vi "String Trim Whitespace.vi"(11 "String":string) -> (3 "*(type *) &x":string)   [LabVIEW 2019]
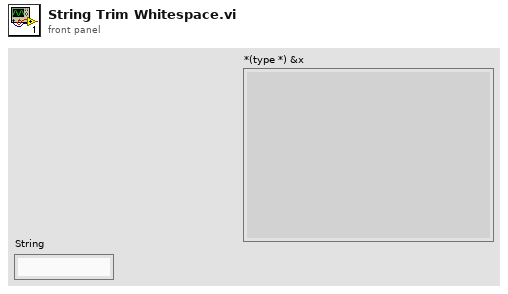
[diagram p1: front panel]
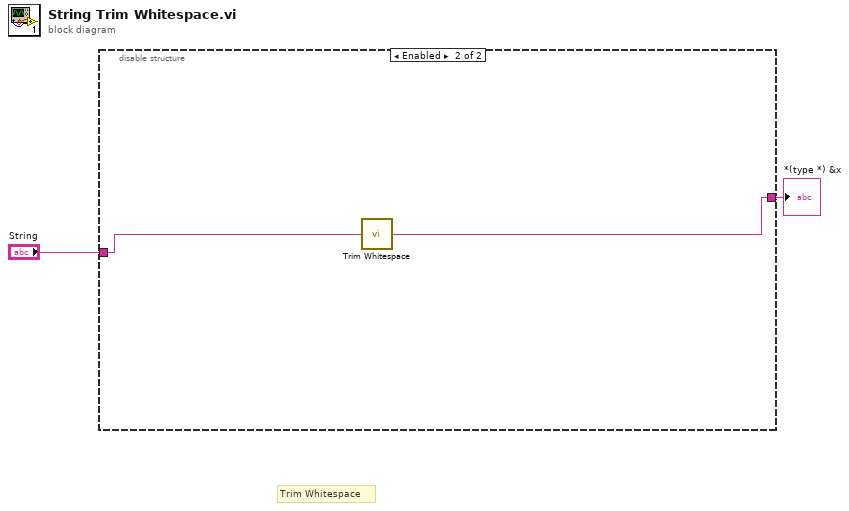
[diagram p0: block diagram]
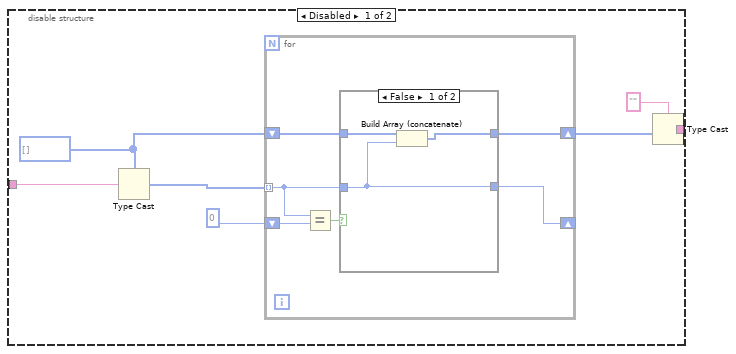
[diagram p2: hidden frame]
diagram:
  # "Trim Whitespace"
  n1 = disable-structure shown="Enabled" {
    disable-tunnel: [w4 w21] -> w2
    disable-tunnel: "String" -> [w3 w22]
    frame Disabled {
      w7 = u8[] []
      n2 = Type Cast(type=w7, x=w3) -> (*(type *) &x=w9:u8[])
      n3 = for {
        tunnel: w9 -> [w11] mode=indexing
        shift-right: [w10] -> _
        shift-left: u8 0 -> [w15]
        shift-right: [w12] -> w5
        shift-left: w7 -> [w13]
        n4 = Equal?(x=w11, y=w15) -> (x = y?=w14:bool)
        n5 = case shown="False" w14 {
          tunnel: w13 -> [w18 w20]
          tunnel: [w17 w20] -> w12
          tunnel: w11 -> [w16 w19]
          tunnel: [w16 w19] -> w10
          frame False {
            n6 = Build Array (concatenate)(w18, w16) -> (w17:u8[])
          }
          frame True {
          }
        }
      }
      n7 = Type Cast(type="", x=w5) -> (*(type *) &x=w4:string)
    }
    frame Enabled {
      n8 = call <vilib>:"Trim Whitespace.vi"("string"=w22) -> ("trimmed string"=w21:string)  [unwired: 1 in]
    }
  }
  "*(type *) &x" <- w2
